vi "Pulse and Clock Generation.vi"() -> ()   [LabVIEW 2026]
uses:
  <vilib>/Platform/TimedLoop/XDataNode/timing_clust.ctl
  <vilib>/Platform/TimedLoop/XDataNode/nitl_modes.ctl
  <vilib>/Platform/TimedLoop/XDataNode/wakeup.ctl
  <vilib>/rvi/Emulation/niFpgaGetClockAttributes.vi
  <vilib>/rvi/Emulation/niFpgaSctlEmulationGetInTimedLoop.vi
  <vilib>/rvi/Emulation/niFpgaEmulationReportErrorSimple.vi
  <vilib>/rvi/Emulation/niFpgaProcessEmulError.vi
  <vilib>/rvi/Emulation/niFpgaCriticalErrorInLSC.vi
  <vilib>/rvi/eio/common/nirviEmuTemplateMethod_errors.vi
  <vilib>/platform/TimedLoop/XDataNode/XDataNode.xnode
  <vilib>/eio/EIONode/EIONode.xnode
  <vilib>/Platform/TimedLoop/XDataNode/XDNodeRunTimeDep.lvlib
panel:
  in  "Reset":bool=TRUE
  out "Clock Ticks":u32
  out "Output":bool
  in  "Enable Output":bool
  out "Requested Output Ticks":i32
  in  "Requested Output Frequency":sgl=10.0
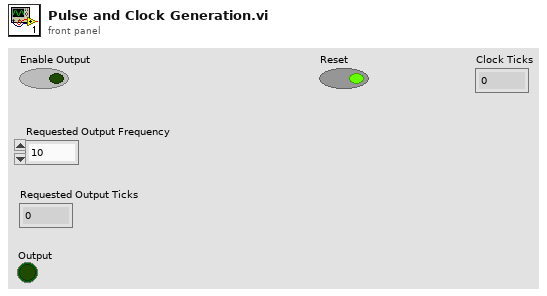
[diagram p1: front panel]
types:
  T1 = typedef "XDNodeRunTimeDep.lvlib/timing_clust.ctl" = cluster{"Expected End [f-1]":u64, "Actual End [f-1]":u64, "Finished Late? [f-1]":bool, "Expected End [i-1]":u64, "Actual End [i-1]":u64, "Finished Late? [i-1]":bool, "Expected Start [i]":u64, "Actual Start [i]":u64, "Expected Start [f]":u64, "Actual Start [f]":u64, "Source Name":string, "Structure Name":string, "Period":i64, "Deadline":i64, "Offset":i64, "Start":i64, "Priority":i32, "Timeout":i32, "Mode":T2, "Wakeup Reason":T3, "Error":errorcluster, "Source Type":string, "Secondary Source Type":string, "Global End Time":u64, "Global Start Time":u64, "Frame Duration":u64, "Iteration Duration":u64, "Assigned CPU":i32, "I/O Scan Engine Mode":u32}
  T2 = typedef "XDNodeRunTimeDep.lvlib/nitl_modes.ctl" = enum32{"No Change", "Process missed periods, maintain original phase", "Discard missed periods, maintain original phase", "Process missed periods, ignore original phase", "Discard missed periods, ignore original phase"}
  T3 = typedef "XDNodeRunTimeDep.lvlib/wakeup.ctl" = enum32{"Normal", "Aborted", "Asynchronous wakeup", "Timing source error", "Timed loop error", "Timeout"}
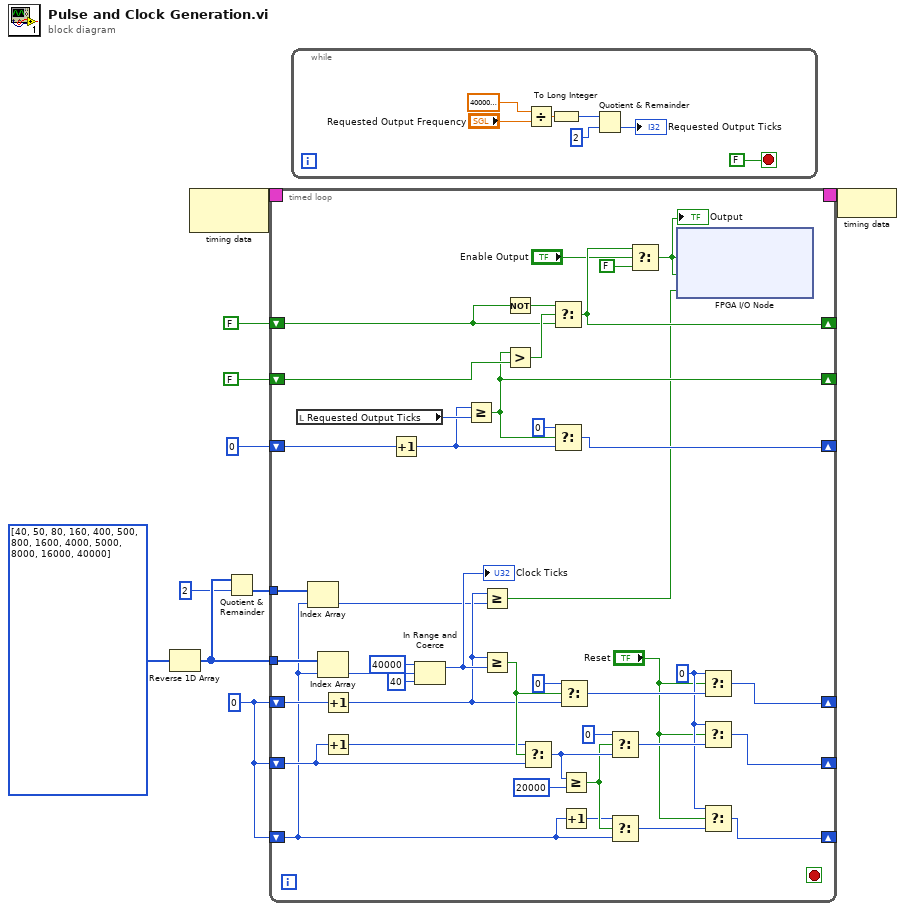
[diagram p0: block diagram]
diagram:
  w4 = u32 0
  n1 = Reverse 1D Array(array=u32[] [40, 50, 80, 160, 400, 500, 800, 1600, 4000, 5000, 8000, 16000, 40000]) -> (reversed array=w3:u32[])
  n2 = node-c288() -> (w10:T1)  [unwired: 1 in]
  n3 = Quotient & Remainder(x=w3, y=i16 2) -> (floor(x/y)=w1:u32[])  [unwired: 1 out]
  n4 = timed-loop {
    timing: w10 -> [_]
    timing-out: [_] -> w9
    shift-right: [w52] -> _
    shift-left: 0 -> [w51]
    shift-right: [w47] -> _
    shift-left: FALSE -> [w48]
    shift-right: [w41] -> _
    shift-left: FALSE -> [w45]
    shift-right: [w18] -> _
    shift-left: w4 -> [w37]
    tunnel: w3 -> [w36]
    shift-right: [w20] -> _
    shift-left: w4 -> [w34]
    shift-right: [w22] -> _
    shift-left: w4 -> [w11]
    tunnel: w1 -> [w14]
    stop <- _ stop-if-true
    w17 = u32 0 ("t")
    n5 = local read "Requested Output Ticks"() -> (w50:i32)
    n6 = Index Array(array=w14, index=w11) -> (element=w13:u32)
    n7 = Index Array(array=w36, index=w11) -> (element=w25:u32)
    n8 = Increment(x=w37) -> (x+1=w15:u32)
    n9 = Increment(x=w34) -> (x+1=w33:u32)
    n10 = Increment(x=w51) -> (x+1=w43:i32)
    n11 = In Range and Coerce(upper limit=u32 40000, x=w25, lower limit=u32 40) -> (coerced(x)=w24:u32)  [unwired: 1 out]
    "Clock Ticks" <- w24
    n12 = Greater Or Equal?(x=w43, y=w50) -> (x >= y?=w47:bool)
    n13 = Greater Or Equal?(x=w15, y=w13) -> (x >= y?=w12:bool)
    n14 = Greater Or Equal?(x=w15, y=w24) -> (x >= y?=w35:bool)
    n15 = Not(x=w45) -> (.not. x?=w44:bool)
    n16 = Greater?(x=w47, y=w48) -> (0:w46:bool)
    n17 = Select(t=w33, s=w35, f=w34) -> (s? t:f=w30:u32)
    n18 = Select(t=w44, s=w46, f=w45) -> (s? t:f=w41:bool)
    n19 = Select(t=0, s=w47, f=w43) -> (s? t:f=w52:i32)
    n20 = Select(t=u32 0, s=w35, f=w15) -> (s? t:f=w19:u32)
    n21 = Greater Or Equal?(x=w30, y=u32 20000) -> (x >= y?=w29:bool)
    n22 = Increment(x=w11) -> (x+1=w28:u32)
    n23 = Select(t=u32 0, s=w29, f=w30) -> (s? t:f=w21:u32)
    n24 = Select(t=w28, s=w29, f=w11) -> (s? t:f=w23:u32)
    n25 = Select(t=w41, s="Enable Output", f=FALSE) -> (s? t:f=w39:bool)
    "Output" <- w39
    n26 = xnode "FPGA I/O Node"("Connector1/DIO0"=w39, "Connector1/DIO1"=w39, "Connector1/DIO2"=w12) -> ()  [unwired: 3 in, 3 out]
    n27 = Select(t=w17, s="Reset", f=w19) -> (s? t:f=w18:u32)
    n28 = Select(t=w17, s="Reset", f=w21) -> (s? t:f=w20:u32)
    n29 = Select(t=w17, s="Reset", f=w23) -> (s? t:f=w22:u32)
  }
  n30 = while {
    stop <- FALSE stop-if-true
    n31 = Divide(x=sgl 40000000.0 ("y"), y="Requested Output Frequency") -> (x/y=w59:sgl)
    n32 = To Long Integer(number=w59) -> (32bit integer=w56:i32)
    n33 = Quotient & Remainder(x=w56, y=2) -> (floor(x/y)=→"Requested Output Ticks":i32)  [unwired: 1 out]
  }
  n34 = node-c288(w9) -> ()
